vi "moveAxisBacklash.vi"(8 "error in (no error)":errorcluster, 10 "Settings":T1, 11 "Current Position":dbl[](array[numeric])) -> (0 "error out":errorcluster)   [LabVIEW 2017]
uses:
  Settings/Settings-Control.ctl
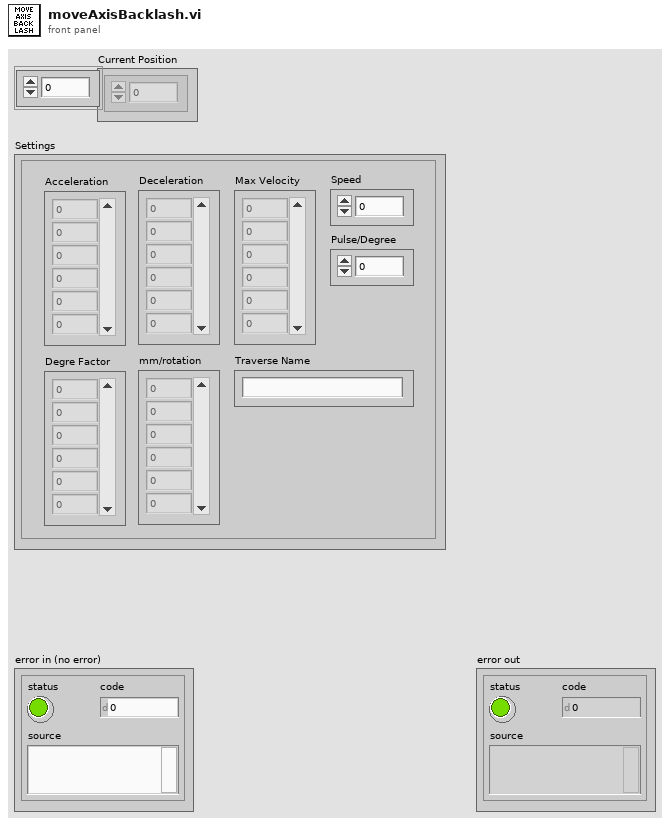
[diagram p1: front panel]
types:
  T1 = typedef "Settings-Control.ctl" = cluster{"Acceleration":dbl[], "Deceleration":dbl[], "Max Velocity":dbl[], "Speed":dbl, "Pulse/Degree":dbl, "Degre Factor":dbl[], "mm/rotation":dbl[], "Traverse Name":string}
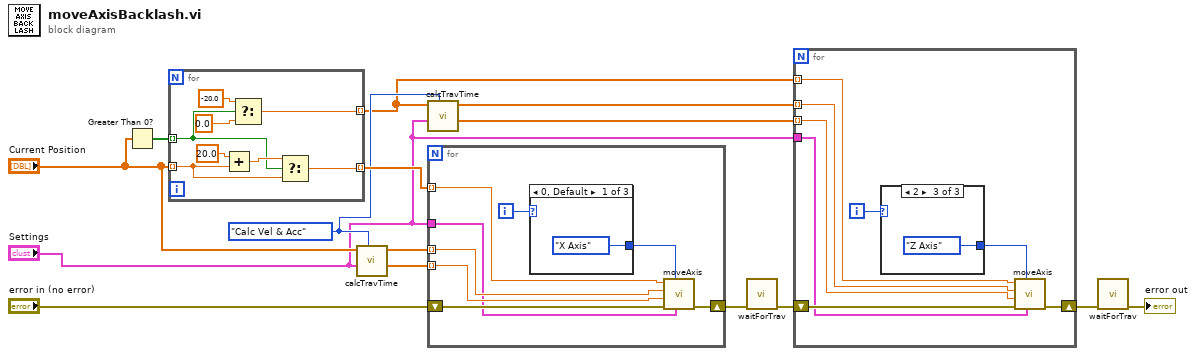
[diagram p0: block diagram]
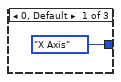
[diagram p2: hidden frame]
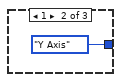
[diagram p3: hidden frame]
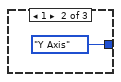
[diagram p4: hidden frame]
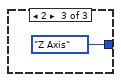
[diagram p5: hidden frame]
diagram:
  w6 = enum16{"Calc Vel & Acc", "Check Time"}."Calc Vel & Acc" ("Mode")
  n1 = Greater Than 0?(x="Current Position") -> (x > 0?=w10:bool[])
  n2 = for {
    tunnel: w10 -> [w17] mode=indexing
    tunnel: "Current Position" -> [w23] mode=indexing
    tunnel: [w20] -> w13 mode=indexing
    tunnel: [w16] -> w1 mode=indexing
    n3 = Add(x=20.0, y=w23) -> (x+y=w22:dbl)
    n4 = Select(t=-20.0 ("x"), s=w17, f=0.0) -> (s? t:f=w16:dbl)
    n5 = Select(t=w22, s=w17, f=w23) -> (s? t:f=w20:dbl)
  }
  n6 = call "calcTravTime.vi"("Mode"=w6, "Settings"="Settings", "Total Distance"="Current Position") -> ("Accelerations"=w8:dbl[], "Velocities"=w7:dbl[])  [unwired: 6 in, 1 out]
  n7 = call "calcTravTime.vi"("Mode"=w6, "Settings"="Settings", "Total Distance"=w1) -> ("Accelerations"=w3:dbl[], "Velocities"=w4:dbl[])  [unwired: 6 in, 1 out]
  n8 = for {
    tunnel: w7 -> [w28] mode=indexing
    tunnel: w8 -> [w31] mode=indexing
    tunnel: "Settings" -> [w26]
    shift-right: [w25] -> w15
    shift-left: "error in (no error)" -> [w29]
    tunnel: w13 -> [w24] mode=indexing
    i -> [w30]
    n9 = case shown="0, Default" w30 {
      tunnel: [enum16{"X Axis", "Y Axis", "Z Axis"}."X Axis" ("Channel") enum16{"X Axis", "Y Axis", "Z Axis"}."Y Axis" ("Channel") enum16{"X Axis", "Y Axis", "Z Axis"}."Z Axis" ("Channel")] -> w27
      frame 0, Default {
      }
      frame 1 {
      }
      frame 2 {
      }
    }
    n10 = call "moveAxis.vi"("Settings"=w26, "Channel"=w27, "error in"=w29, "Acceleration"=w31, "Velocity"=w28, "Position (mm)"=w24) -> ("error out"=w25:errorcluster)  [unwired: 5 in]
  }
  n11 = call "waitForTrav.vi"("error in"=w15) -> ("error out"=w11:errorcluster)  [unwired: 10 in]
  n12 = for {
    tunnel: w4 -> [w39] mode=indexing
    tunnel: w3 -> [w42] mode=indexing
    tunnel: "Settings" -> [w37]
    shift-right: [w36] -> w12
    shift-left: w11 -> [w40]
    tunnel: w1 -> [w35] mode=indexing
    i -> [w41]
    n13 = case shown="2" w41 {
      tunnel: [enum16{"X Axis", "Y Axis", "Z Axis"}."X Axis" ("Channel") enum16{"X Axis", "Y Axis", "Z Axis"}."Y Axis" ("Channel") enum16{"X Axis", "Y Axis", "Z Axis"}."Z Axis" ("Channel")] -> w38
      frame 0, Default {
      }
      frame 1 {
      }
      frame 2 {
      }
    }
    n14 = call "moveAxis.vi"("Settings"=w37, "Channel"=w38, "error in"=w40, "Acceleration"=w42, "Velocity"=w39, "Position (mm)"=w35) -> ("error out"=w36:errorcluster)  [unwired: 5 in]
  }
  n15 = call "waitForTrav.vi"("error in"=w12) -> ("error out"=→"error out":errorcluster)  [unwired: 10 in]
